vi "Table, Save to Spreadsheet.vi"(5 "append to file (F)":bool, 6 "error in":errorcluster, 8 "spreadsheet file":path=path "C:/ATS Reports/results.txt", 9 "Tbl Refnum":refnum<vi>) -> (0 "error out":errorcluster, 3 "Tbl Refnum dup":refnum<vi>)   [LabVIEW 2010]
doc: "This function saves a table to a spreadsheet file."
uses:
  <vilib>/Utility/file.llb/Write To Spreadsheet File (string).vi
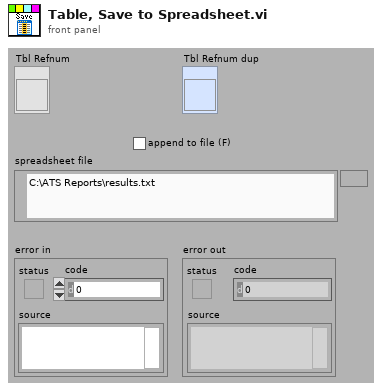
[diagram p1: front panel]
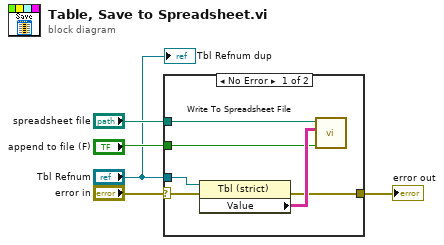
[diagram p0: block diagram]
diagram:
  n1 = case shown="No Error" "error in" {
    selector: "error in" -> [w10 w12]
    tunnel: [w9 w12] -> w5
    tunnel: "spreadsheet file" -> [w8 _]
    tunnel: "append to file (F)" -> [w7 _]
    tunnel: "Tbl Refnum" -> [w6 _]
    frame No Error {
      n2 = property class="Tbl (strict)"(reference=w6, error in=w10) -> (error out=w9:errorcluster, "Value"=w11:string[][])  [unwired: 1 out]
      n3 = call-poly <vilib>:"Write To Spreadsheet File.vi"("append to file? (new file:F)"=w7, "2D data"=w11, "file path (dialog if empty)"=w8) -> ()  [unwired: 5 in, 1 out]
    }
    frame Error {
    }
  }
  "error out" <- w5
  "Tbl Refnum dup" <- "Tbl Refnum"
